vi "DP-Extract Comparisons.vi"(0 "Comparison list":T2, 7 "Criterion":dbl, 9 "F2 (kHz)":dbl, 11 "Which DP":enum16{"2f1-f2", "f2-f1"}(ring)) -> (4 "DP Plots":cluster{"F2 array":dbl[], "DPGram":dbl[]}[](array[cluster]), 6 "Names":string[](array[string]), 10 "IO Plots":T1(array[cluster]), 15 "Noise floor data":dbl[][](array[numeric]))   [LabVIEW 2020]
uses:
  Typedefs/DP-Comparison List.ctl
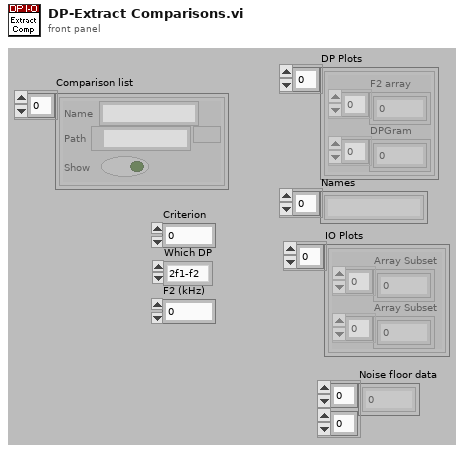
[diagram p1: front panel]
types:
  T1 = cluster{"Array Subset":dbl[], "Array Subset":dbl[]}[]
  T2 = typedef "DP-Comparison List.ctl" = cluster{"Name":string, "Path":path, "Show":bool}[]
  T3 = cluster{"Array Subset":dbl[], "Array Subset":dbl[]}
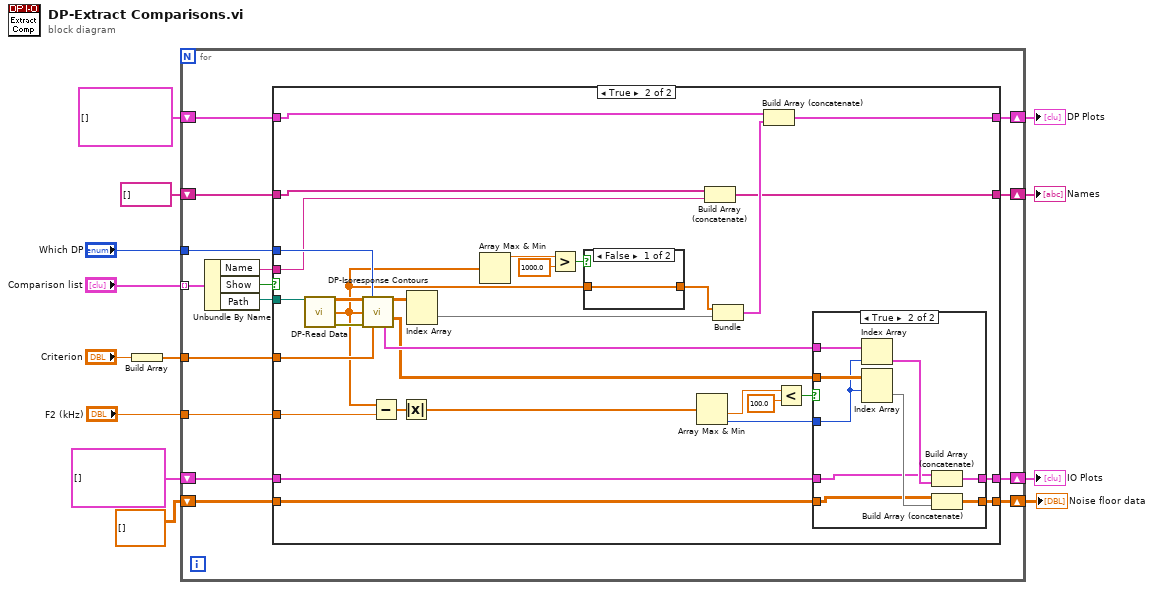
[diagram p0: block diagram]
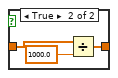
[diagram p3: hidden frame]
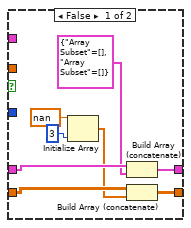
[diagram p4: hidden frame]
diagram:
  n1 = Build Array("Criterion") -> (w11:dbl[])
  n2 = for {
    tunnel: "Comparison list" -> [w28] mode=indexing
    tunnel: "Which DP" -> [w26]
    tunnel: w11 -> [w25]
    shift-right: [w23] -> w7
    shift-left: cluster{"F2 array":dbl[], "DPGram":dbl[]}[] [] -> [w22]
    shift-right: [w20] -> w6
    shift-left: string[] [] -> [w19]
    tunnel: "F2 (kHz)" -> [w18]
    shift-right: [w17] -> w2
    shift-left: T1 [] -> [w15]
    shift-right: [w16] -> w1
    shift-left: dbl[][] [] -> [w14]
    n3 = Unbundle By Name(w28) -> ("Name"=w21:string, "Show"=w24:bool, "Path"=w27:path)
    n4 = case shown="True" w24 {
      tunnel: w27 -> [_ w61]
      tunnel: w26 -> [_ w60]
      tunnel: w25 -> [_ w59]
      tunnel: [w32 w55] -> w23
      tunnel: w22 -> [w32 w54]
      tunnel: w21 -> [_ w53]
      tunnel: [w31 w52] -> w20
      tunnel: w19 -> [w31 w51]
      tunnel: w18 -> [_ w50]
      tunnel: [w30 w42] -> w17
      tunnel: [w29 w41] -> w16
      tunnel: w15 -> [w30 w40]
      tunnel: w14 -> [w29 w39]
      frame False {
      }
      frame True {
        n5 = call "DP-Read Data.vi"("Path"=w61) -> ("Data matrix"=w62:dbl[][], "F2 array"=w35:dbl[], "error out"=w63:errorcluster)  [unwired: 11 in, 1 out]
        n6 = call "DP-Isoresponse Contours.vi"("Data matrix"=w62, "Which DP"=w60, "F2 array"=w35, "error in"=w63, "criteria (dB)"=w59) -> ("DPGram"=w58:dbl[][], "Noise floor data"=w33:dbl[][], "IO Functions"=w43:T1)  [unwired: 5 in, 3 out]
        n7 = Subtract(x=w35, y=w50) -> (x-y=w49:dbl[])
        n8 = Absolute Value(x=w49) -> (abs(x)=w48:dbl[])
        n9 = Index Array(array=w58) -> (element=w57:dbl[])  [unwired: 2 in]
        n10 = Array Max & Min(array=w35) -> (max value=w36:dbl)  [unwired: 3 out]
        n11 = Greater?(x=w36, y=1000.0) -> (0:w38:bool)
        n12 = case shown="False" w38 {
          tunnel: [w64 w67] -> w34
          tunnel: w35 -> [w64 w65]
          frame False {
          }
          frame True {
            n13 = Divide(x=w65, y=1000.0) -> (x/y=w67:dbl[])
          }
        }
        n14 = Array Max & Min(array=w48) -> (min value=w47:dbl, min index (indices)=w44:i32)  [unwired: 2 out]
        n15 = Build Array (concatenate)(w51, w53) -> (w52:string[])
        n16 = Bundle("F2 array"=w34, "DPGram"=w57) -> (w56:cluster{"F2 array":dbl[], "DPGram":dbl[]})  [unwired: 1 in]
        n17 = Build Array (concatenate)(w54, w56) -> (w55:cluster{"F2 array":dbl[], "DPGram":dbl[]}[])
        n18 = Less?(x=w47, y=100.0) -> (x < y?=w45:bool)
        n19 = case shown="True" w45 {
          tunnel: w44 -> [_ w82]
          tunnel: w33 -> [_ w84]
          tunnel: w43 -> [_ w83]
          tunnel: [w75 w79] -> w42
          tunnel: [w74 w78] -> w41
          tunnel: w40 -> [w73 w77]
          tunnel: w39 -> [w72 w76]
          frame False {
            n20 = Initialize Array(nan ("element"), 3 ("dimension size")) -> (w68:dbl[])
            n21 = Build Array (concatenate)(w73, T3 {"Array Subset"=[], "Array Subset"=[]}) -> (w75:T1)
            n22 = Build Array (concatenate)(w72, w68) -> (w74:dbl[][])
          }
          frame True {
            n23 = Index Array(array=w83, index=w82) -> (element=w81:T3)
            n24 = Index Array(array=w84, index (row)=w82) -> (element=w80:dbl[])  [unwired: 1 in]
            n25 = Build Array (concatenate)(w77, w81) -> (w79:T1)
            n26 = Build Array (concatenate)(w76, w80) -> (w78:dbl[][])
          }
        }
      }
    }
  }
  "DP Plots" <- w7
  "Names" <- w6
  "IO Plots" <- w2
  "Noise floor data" <- w1
